vi "Teleop.vi"(10 "Match Info":T1={"Autonomous Elapsed Seconds"=0.0, "TeleOp Elapsed Seconds"=0.0, "Disabled Elapsed Seconds"=0.0, "Visited Autonomous"=FALSE, "Visited TeleOp"=FALSE, "Visited Disabled"=FALSE, "Autonomous Settings"={"Autonomous Style"=enum."Independent", "VI Refnum"=refnum}}, 11 "Call Context":T2) -> ()   [LabVIEW 2017]
doc: "This VI is called for each TeleOp packet received from the DS where the robot is not disabled. It is often used to read from the joysticks and update I/O or to update setpoints for timed control loops. It should complete and return within 20 milliseconds or it may miss DS packets."
uses:
  <vilib>/Rock Robotics/WPI/DriverStation/WPI_DriverStationDerivedRobotMode.ctl
  <vilib>/Rock Robotics/WPI/DriverStation/WPI_DriverStationMatch Info.ctl
  <vilib>/Rock Robotics/WPI/ThirdParty/Phoenix-LabVIEW/Motor Controller/Controls/CTRE_Phoenix_MotorControl_ControlMode.ctl
  <vilib>/Rock Robotics/WPI/Utilities/WPI_GetSetVariantRefNum.vi
  <vilib>/Rock Robotics/Network Tables/NT Write Numeric Array.vi
  <vilib>/Rock Robotics/WPI/ThirdParty/Phoenix-LabVIEW/Motor Controller/Get/CTRE_Phoenix_MotorController_GetQuadratureData.vi
  <vilib>/Rock Robotics/Network Tables/NT Read Numeric Array.vi
  <vilib>/Rock Robotics/Network Tables/NT Write Number.vi
  <vilib>/Rock Robotics/WPI/Solenoid/Deprecated/WPI_SolenoidSetBool.vi
  <vilib>/Rock Robotics/Network Tables/NT Read Boolean.vi
  <vilib>/Rock Robotics/Network Tables/NT Read Number.vi
panel:
  out "Sample Slider 0":dbl(slide) scale=0.0..5.0
  out "Sample Boolean 1":bool
  out "Sample Boolean 0":bool
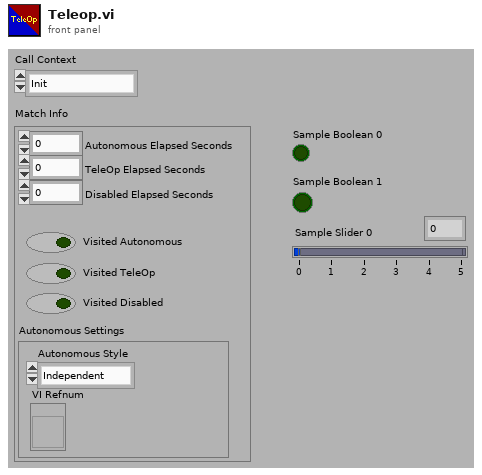
[diagram p1: front panel]
types:
  T1 = typedef "WPI_DriverStationMatch Info.ctl" = cluster{"Autonomous Elapsed Seconds":dbl, "TeleOp Elapsed Seconds":dbl, "Disabled Elapsed Seconds":dbl, "Visited Autonomous":bool, "Visited TeleOp":bool, "Visited Disabled":bool, "Autonomous Settings":cluster{"Autonomous Style":enum16{"Iterative", "Independent"}, "VI Refnum":refnum<vi>}}
  T2 = typedef "WPI_DriverStationDerivedRobotMode.ctl" = enum16{"Init", "Execute", "Stop"}
  T3 = typedef "CTRE_Phoenix_MotorControl_ControlMode.ctl" = u16
  T4 = typedef "WPI_MotorControlDeviceRef.ctl" = cluster{"DeviceStatus":errorcluster, "Type":T5, "PWM":cluster{"PWM Channel":T6, "DeadBand":T7}, "CAN":cluster{"Device Number":u8, "SetOutput VI Ref":variant, "GetOutput VI Ref":variant, "Enable VI Ref":variant, "Disable VI Ref":variant, "Data":variant}, "Invert":bool, "DIO PWM":cluster{"PWM \"Enable\" Channel":T6, "DIOChannel":T8, "PWM Rate":dbl}}
  T5 = typedef "WPI_MotorControlType.ctl" = enum16{"PWM", "CAN", "DIO PWM"}
  T6 = typedef "FPGA_DIOPWMChannel.ctl" = enum8{"PWM 0", "PWM 1", "PWM 2", "PWM 3", "PWM 4", "PWM 5", "PWM 6", "PWM 7", "PWM 8", "PWM 9", "PWM MXP 0", "PWM MXP 1", "PWM MXP 2", "PWM MXP 3", "PWM MXP 4", "PWM MXP 5", "PWM MXP 6", "PWM MXP 7", "PWM MXP 8", "PWM MXP 9", "Invalid"}
  T7 = typedef "WPI_PWMDeadband.ctl" = cluster{"Name":string, "maxPositivePwm":i32, "minPositivePwm":i32, "centerPwm":i32, "maxNegativePwm":i32, "minNegativePwm":i32, "angularRange":u16}
  T8 = typedef "FPGA_DIOChannel.ctl" = enum8{"DIO 0", "DIO 1", "DIO 2", "DIO 3", "DIO 4", "DIO 5", "DIO 6", "DIO 7", "DIO 8", "DIO 9", "DIO MXP 0", "DIO MXP 1", "DIO MXP 2", "DIO MXP 3", "DIO MXP 4", "DIO MXP 5", "DIO MXP 6", "DIO MXP 7", "DIO MXP 8", "DIO MXP 9", "DIO MXP 10", "DIO MXP 11", "DIO MXP 12", "DIO MXP 13", "DIO MXP 14", "DIO MXP 15", "SPI Port CS1", "SPI Port CS2", "SPI Port CS3", "SPI Port MISO", "SPI Port MOSI", "Invalid"}
  T9 = typedef "WPI_JoystickDevRef.ctl" = cluster{"Device":T10}
  T10 = typedef "WPI_JoystickDeviceEnum.ctl" = enum16{"USB 0", "USB 1", "USB 2", "USB 3", "USB 4", "USB 5"}
  T11 = typedef "WPI_RobotDriveDevRef.ctl" = cluster{"DevStatus":errorcluster, "Motors[]":T4[], "Square Inputs":bool, "Max Output":dbl}
  T12 = typedef "WPI_CompressorDevRef.ctl" = cluster{"DevStatus":errorcluster, "Pneumatics Control Module":u8}
  T13 = typedef "WPI_SolenoidDevRef.ctl" = cluster{"DevStatus":errorcluster, "Pneumatics Control Module":u8, "Forward Solenoid Channel":T14, "Reverse Solenoid Channel":T14}
  T14 = typedef "WPI_SolenoidChannel.ctl" = enum8{"Solenoid 0", "Solenoid 1", "Solenoid 2", "Solenoid 3", "Solenoid 4", "Solenoid 5", "Solenoid 6", "Solenoid 7", "Invalid"}
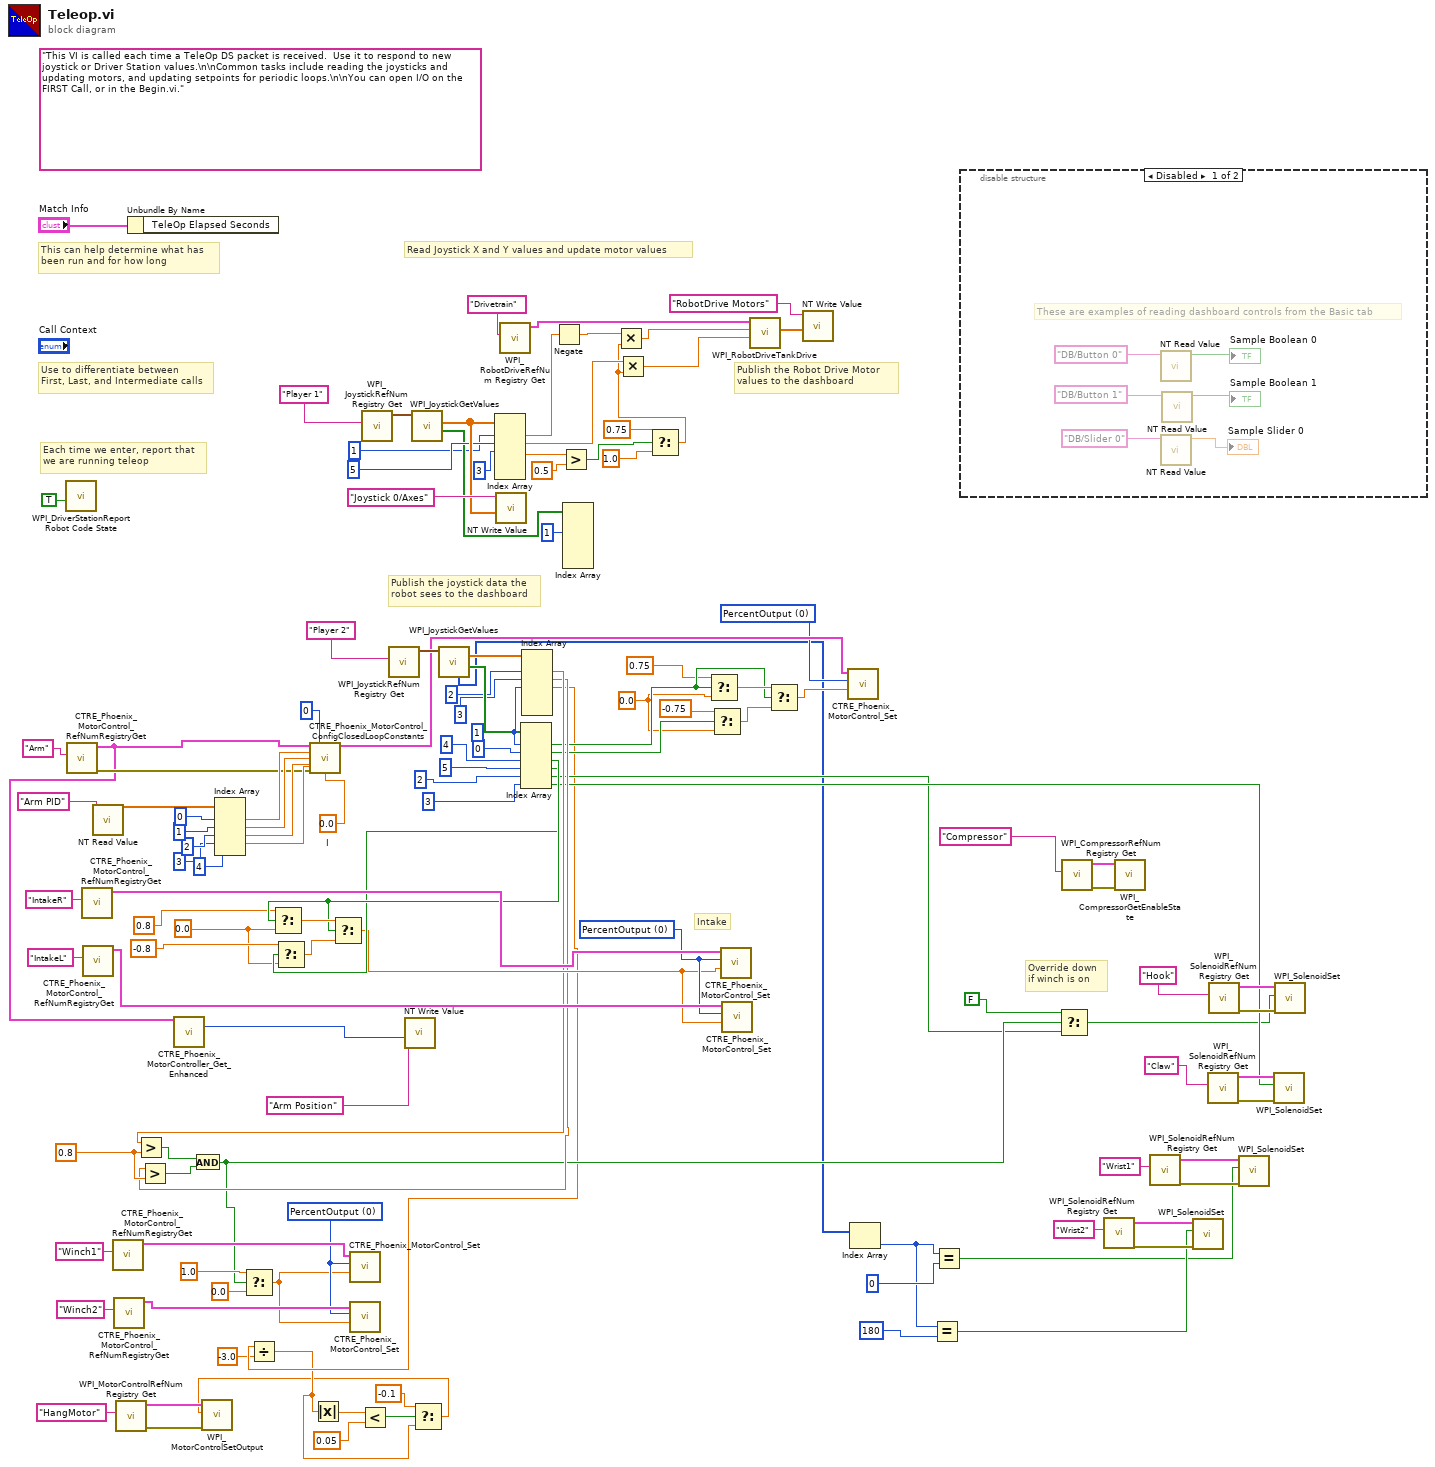
[diagram p0: block diagram]
diagram:
  w41 = 0.0 ("t")
  w7 = 1 ("index")
  w49 = T3 0 items=["PercentOutput"=0, "Position"=1, "Velocity"=2, "Current"=3, "Follower"=5, "MotionProfile"=6, "MotionMagic"=7, "MotionMagicArc"=8, "MotionProfileArc"=10, "Disabled"=15] ("Control Mode")
  w57 = 0.8 ("y")
  w63 = T3 0 items=["PercentOutput"=0, "Position"=1, "Velocity"=2, "Current"=3, "Follower"=5, "MotionProfile"=6, "MotionMagic"=7, "MotionMagicArc"=8, "MotionProfileArc"=10, "Disabled"=15] ("Control Mode")
  w65 = 0.0
  w74 = T3 0 items=["PercentOutput"=0, "Position"=1, "Velocity"=2, "Current"=3, "Follower"=5, "MotionProfile"=6, "MotionMagic"=7, "MotionMagicArc"=8, "MotionProfileArc"=10, "Disabled"=15] ("Control Mode")
  w118 = 0.0  # I
  (unwired) "This VI is called each time a TeleOp DS packet is received.  Use it to respond to new joystick or Driver Station values.\n\nCommon tasks include reading the joysticks and updating motors, and updating setpoints for periodic loops.\n\nYou can open I/O on the FIRST Call, or in the Begin.vi."
  # "Override down\nif winch is on"
  # "Intake"
  # "Publish the Robot Drive Motor\nvalues to the dashboard"
  # "Publish the joystick data the\nrobot sees to the dashboard"
  # "Each time we enter, report that\nwe are running teleop"
  # "Use to differentiate between\nFirst, Last, and Intermediate calls"
  # "This can help determine what has\nbeen run and for how long"
  # "Read Joystick X and Y values and update motor values"
  n1 = call <vilib>:"WPI_DriverStationReport Robot Code State.vi"("TeleOp"=TRUE ("Autonomous")) -> ()  [unwired: 10 in, 1 out]
  n2 = call <vilib>:"CTRE_Phoenix_MotorControl_RefNumRegistryGet.vi"("refnum name"="Arm") -> ("error out"=w78:errorcluster, "PhoenixMotorControlDevRef"=w77:T4)  [unwired: 9 in]
  n3 = call <vilib>:"CTRE_Phoenix_MotorControl_RefNumRegistryGet.vi"("refnum name"="IntakeR") -> ("PhoenixMotorControlDevRef"=w109:T4)  [unwired: 9 in, 1 out]
  n4 = call <vilib>:"CTRE_Phoenix_MotorControl_RefNumRegistryGet.vi"("refnum name"="IntakeL") -> ("PhoenixMotorControlDevRef"=w110:T4)  [unwired: 9 in, 1 out]
  n5 = call-poly <vilib>:"NT Read Value.vi"("Name"="Arm PID") -> ("Numeric Array"=w88:dbl[])  [unwired: 9 in, 1 out]
  n6 = call <vilib>:"CTRE_Phoenix_MotorControl_RefNumRegistryGet.vi"("refnum name"="Winch1") -> ("PhoenixMotorControlDevRef"=w106:T4)  [unwired: 9 in, 1 out]
  n7 = call <vilib>:"CTRE_Phoenix_MotorControl_RefNumRegistryGet.vi"("refnum name"="Winch2") -> ("PhoenixMotorControlDevRef"=w105:T4)  [unwired: 9 in, 1 out]
  n8 = call <vilib>:"WPI_MotorControlRefNum Registry Get.vi"("refnum name"="HangMotor") -> ("error out"=w35:errorcluster, "MotorControlDevRef"=w36:T4)  [unwired: 9 in]
  n9 = Unbundle By Name("Match Info") -> ()  [unwired: 1 out]
  n10 = call-poly <vilib>:"CTRE_Phoenix_MotorController_Get_Enhanced.vi"("PhoenixMotorControlDevRef"=w77) -> ("Quadrature Position"=w76:i32)  [unwired: 11 in, 3 out]
  n11 = Index Array(array=w88, index #1=0 ("index"), index #2=1 ("index"), index #3=2 ("index"), index #4=3 ("index"), index #5=4 ("index")) -> (element #1=w83:dbl, element #2=w82:dbl, element #3=w81:dbl, element #4=w80:dbl)  [unwired: 1 out]
  n12 = call <vilib>:"CTRE_Phoenix_MotorControl_ConfigClosedLoopConstants.vi"("PhoenixMotorControlDevRef"=w77, "slotIdx"=0, "P"=w83, "I"=w82, "D"=w81, "error in (no error)"=w78, "F"=w80, "I Zone"=w118) -> ("PhoenixMotorControlDevRef"=w90:T4)  [unwired: 6 in, 1 out]
  n13 = call <vilib>:"WPI_JoystickRefNum Registry Get.vi"("refnum name"="Player 1") -> ("JoystickDevRef"=w126:T9)  [unwired: 1 in, 9 out]
  n14 = call <vilib>:"WPI_JoystickRefNum Registry Get.vi"("refnum name"="Player 2") -> ("JoystickDevRef"=w115:T9)  [unwired: 1 in, 9 out]
  n15 = call-poly <vilib>:"NT Write Value.vi"("Numeric"=w76, "Name"="Arm Position") -> ()  [unwired: 9 in, 1 out]
  n16 = call <vilib>:"WPI_JoystickGetValues.vi"("JoystickDevRef"=w126) -> ("Buttons"=w93:bool[], "Axes"=w123:dbl[])  [unwired: 6 in, 3 out]
  n17 = call <vilib>:"WPI_JoystickGetValues.vi"("JoystickDevRef"=w115) -> ("Buttons"=w113:bool[], "Axes"=w116:dbl[], "POVs"=w13:i16[])  [unwired: 6 in, 2 out]
  n18 = Index Array(array=w123, index #1=1, index #2=5, index #3=3 ("index")) -> (element #1=w95:dbl, element #2=w29:dbl, element #3=w24:dbl)  [unwired: 3 in, 3 out]
  n19 = call-poly <vilib>:"NT Write Value.vi"("Numeric Array"=w123, "Name"="Joystick 0/Axes") -> ()  [unwired: 9 in, 1 out]
  n20 = call <vilib>:"WPI_RobotDriveRefNum Registry Get.vi"("refnum name"="Drivetrain") -> ("RobotDriveDevRef"=w121:T11)  [unwired: 1 in, 9 out]
  n21 = Index Array(array=w113, index #1=w7, index #2=0 ("index"), index #3=4 ("index"), index #4=5 ("index"), index #5=2 ("index"), index #6=3 ("index")) -> (element #1=w45:bool, element #2=w44:bool, element #3=w71:bool, element #4=w70:bool, element #5=w38:bool, element #6=w52:bool)
  n22 = Select(t=0.8, s=w71, f=w65) -> (s? t:f=w73:dbl)
  n23 = Select(t=-0.8, s=w70, f=w65) -> (s? t:f=w72:dbl)
  n24 = Select(t=w73, s=w71, f=w72) -> (s? t:f=w64:dbl)
  n25 = Index Array(array=w116, index #1=2 ("index"), index #2=3 ("index"), index #3=w7) -> (element #1=w56:dbl, element #2=w55:dbl, element #3=w32:dbl)  [unwired: 3 in, 3 out]
  n26 = Greater?(x=w56, y=w57) -> (0:w62:bool)
  n27 = Greater?(x=w55, y=w57) -> (0:w61:bool)
  n28 = And(x=w62, y=w61) -> (x .and. y?=w40:bool)
  n29 = Select(t=1.0, s=w40, f=0.0) -> (s? t:f=w60:dbl)
  n30 = Divide(x=w32, y=-3.0) -> (x/y=w2:dbl)
  n31 = Absolute Value(x=w2) -> (abs(x)=w6:dbl)
  n32 = call <vilib>:"CTRE_Phoenix_MotorControl_Set.vi"("Output"=w60, "Control Mode"=w63, "PhoenixMotorControlDevRef"=w106) -> ()  [unwired: 7 in, 2 out]
  n33 = call <vilib>:"CTRE_Phoenix_MotorControl_Set.vi"("Output"=w60, "Control Mode"=w63, "PhoenixMotorControlDevRef"=w105) -> ()  [unwired: 7 in, 2 out]
  n34 = Less?(x=w6, y=0.05) -> (x < y?=w4:bool)
  n35 = Select(t=-0.1, s=w4, f=w2) -> (s? t:f=w1:dbl)
  n36 = call <vilib>:"WPI_MotorControlSetOutput.vi"("error in (no error)"=w35, "Output"=w1, "MotorControlDevRef"=w36) -> ()  [unwired: 6 in, 3 out]
  n37 = Negate(x=w95) -> (-x=w30:dbl)
  n38 = Greater?(x=w24, y=0.5) -> (0:w22:bool)
  n39 = Index Array(array=w93, index #2=1 ("index")) -> ()  [unwired: 5 in, 6 out]
  n40 = Select(t=0.75, s=w22, f=1.0) -> (s? t:f=w20:dbl)
  n41 = Multiply(x=w30, y=w20) -> (x*y=w27:dbl)
  n42 = Multiply(x=w29, y=w20) -> (x*y=w26:dbl)
  n43 = Select(t=0.75, s=w45, f=w41) -> (s? t:f=w48:dbl)
  n44 = Select(t=-0.75, s=w44, f=w41) -> (s? t:f=w47:dbl)
  n45 = call <vilib>:"CTRE_Phoenix_MotorControl_Set.vi"("Output"=w64, "Control Mode"=w74, "PhoenixMotorControlDevRef"=w109) -> ()  [unwired: 7 in, 2 out]
  n46 = call <vilib>:"CTRE_Phoenix_MotorControl_Set.vi"("Output"=w64, "Control Mode"=w74, "PhoenixMotorControlDevRef"=w110) -> ()  [unwired: 7 in, 2 out]
  n47 = call <vilib>:"WPI_RobotDriveTankDrive.vi"("Right axis value"=w26, "Left axis value"=w27, "RobotDriveDevRef"=w121) -> ("Motor Values"=w120:dbl[])  [unwired: 6 in, 2 out]
  n48 = Select(t=w48, s=w45, f=w47) -> (s? t:f=w46:dbl)
  n49 = call-poly <vilib>:"NT Write Value.vi"("Numeric Array"=w120, "Name"="RobotDrive Motors") -> ()  [unwired: 9 in, 1 out]
  n50 = call <vilib>:"CTRE_Phoenix_MotorControl_Set.vi"("Output"=w46, "Control Mode"=w49, "PhoenixMotorControlDevRef"=w90) -> ()  [unwired: 7 in, 2 out]
  n51 = Index Array(array=w13) -> (element=w11:i16)  [unwired: 1 in]
  n52 = Equal?(x=w11, y=180) -> (x = y?=w9:bool)
  n53 = Equal?(x=w11, y=0) -> (x = y?=w8:bool)
  n54 = disable-structure shown="Disabled" {
    frame Disabled {
      # "These are examples of reading dashboard controls from the Basic tab"
      n55 = call-poly <vilib>:"NT Read Value.vi"("Name"="DB/Button 0" ("refnum name")) -> ("Boolean"=→"Sample Boolean 0":bool)  [unwired: 9 in, 1 out]
      n56 = call-poly <vilib>:"NT Read Value.vi"("Name"="DB/Slider 0" ("refnum name")) -> ("Numeric"=→"Sample Slider 0":dbl)  [unwired: 9 in, 1 out]
      n57 = call-poly <vilib>:"NT Read Value.vi"("Name"="DB/Button 1" ("refnum name")) -> ("Boolean"=→"Sample Boolean 1":bool)  [unwired: 9 in, 1 out]
    }
    frame Enabled {
    }
  }
  n58 = Select(t=FALSE, s=w40, f=w38) -> (s? t:f=w37:bool)
  n59 = call <vilib>:"WPI_CompressorRefNum Registry Get.vi"("refnum name"="Compressor") -> ("error out"=w104:errorcluster, "CompressorDevRef"=w103:T12)  [unwired: 9 in]
  n60 = call <vilib>:"WPI_SolenoidRefNum Registry Get.vi"("refnum name"="Wrist2") -> ("error out"=w15:errorcluster, "SolenoidDevRef"=w16:T13)  [unwired: 9 in]
  n61 = call <vilib>:"WPI_CompressorGetEnableState.vi"("error in (no error)"=w104, "CompressorDevRef"=w103) -> ()  [unwired: 6 in, 4 out]
  n62 = call <vilib>:"WPI_SolenoidRefNum Registry Get.vi"("refnum name"="Wrist1") -> ("error out"=w18:errorcluster, "SolenoidDevRef"=w19:T13)  [unwired: 9 in]
  n63 = call-poly <vilib>:"WPI_SolenoidSet.vi"("error in (no error)"=w15, "Value"=w9, "SolenoidDevRef"=w16) -> ()  [unwired: 7 in, 2 out]
  n64 = call <vilib>:"WPI_SolenoidRefNum Registry Get.vi"("refnum name"="Claw") -> ("error out"=w98:errorcluster, "SolenoidDevRef"=w99:T13)  [unwired: 9 in]
  n65 = call <vilib>:"WPI_SolenoidRefNum Registry Get.vi"("refnum name"="Hook") -> ("error out"=w101:errorcluster, "SolenoidDevRef"=w100:T13)  [unwired: 9 in]
  n66 = call-poly <vilib>:"WPI_SolenoidSet.vi"("error in (no error)"=w18, "Value"=w8, "SolenoidDevRef"=w19) -> ()  [unwired: 7 in, 2 out]
  n67 = call-poly <vilib>:"WPI_SolenoidSet.vi"("error in (no error)"=w98, "Value"=w52, "SolenoidDevRef"=w99) -> ()  [unwired: 7 in, 2 out]
  n68 = call-poly <vilib>:"WPI_SolenoidSet.vi"("error in (no error)"=w101, "Value"=w37, "SolenoidDevRef"=w100) -> ()  [unwired: 7 in, 2 out]
